vi "CreatePDF XYGraph.vi"(0 "RedPressure":dbl, 1 "BluePressure":dbl, 2 "Print":bool=TRUE, 3 "Blue Graph Refnum":refnum<vi>, 4 "Red Graph Refnum":refnum<vi>) -> ()   [LabVIEW 2013, in "main.lvlib"]
uses:
  main.lvlib
  <userlib>/Exaprom PDF/Controls/Page setup.ctl
  <userlib>/Exaprom PDF/Controls/Page size.ctl
  <userlib>/Exaprom PDF/Controls/Page Orientation.ctl
  <userlib>/Exaprom PDF/Controls/Page Layout Custom.ctl
  <userlib>/Exaprom PDF/Controls/Page margins.ctl
  <userlib>/Exaprom PDF/Controls/PDF Details.ctl
  <userlib>/Exaprom PDF/Controls/Unit.ctl
  <userlib>/Exaprom PDF/Controls/Font cluster.ctl
  <userlib>/Exaprom PDF/Controls/Font size.ctl
  <userlib>/Exaprom PDF/Controls/Font color.ctl
  <userlib>/Exaprom PDF/Controls/Paragraphe cluster.ctl
  <userlib>/Exaprom PDF/Controls/Texte alignement.ctl
  <userlib>/Exaprom PDF/Controls/Line spacing.ctl
  <userlib>/Exaprom PDF/Controls/Image alignment and position.ctl
  <userlib>/Exaprom PDF/Controls/Image aligment.ctl
panel:
  out "error out":errorcluster
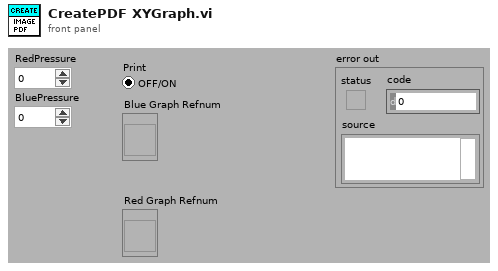
[diagram p1: front panel]
types:
  T1 = typedef "Paragraphe cluster.ctl" = cluster{" Aligment":T2, "Line spacing":T3}
  T2 = typedef "Texte alignement.ctl" = enum16{"Select", "CENTER", "JUSTIFY", "LEFT", "RIGHT"}
  T3 = typedef "Line spacing.ctl" = enum16{"Select", "1.0", "1.5", "2.0"}
  T4 = typedef "Image alignment and position.ctl" = cluster{"Alignment":T5, "X ":sgl, "Y":sgl, "Indentation":sgl}
  T5 = typedef "Image aligment.ctl" = enum16{"Absolute (X,Y) in mm", "Left", "Center", "Right", "Left (textwrap)", "Right (textwrap)"}
  T6 = typedef "Font cluster.ctl" = cluster{"Name":string, "Size":T7, "Color":T8, "Style":cluster{"Bold":bool, "Italic":bool, "Underline":bool, "Strikeout":bool}}
  T7 = typedef "Font size.ctl" = sgl
  T8 = typedef "Font color.ctl" = u32
  T9 = typedef "Unit.ctl" = enum16{"inch", "mm"}
  T10 = typedef "PDF Details.ctl" = cluster{"Title":string, "Subject":string, "Keywords":string, "Author":string, "Creator":string}
  T11 = typedef "Page setup.ctl" = cluster{"Page Size":T12, "Orientation":T13, "Custom Layout":T14, "Margins":T15}
  T12 = typedef "Page size.ctl" = i32
  T13 = typedef "Page Orientation.ctl" = enum16{"Portrait", "Landscape"}
  T14 = typedef "Page Layout Custom.ctl" = cluster{"Width":sgl, "Height":sgl}
  T15 = typedef "Page margins.ctl" = cluster{"Left":sgl, "Right":sgl, "Top":sgl, "Bottom":sgl}
  T16 = typedef "Page dimensions.ctl" = cluster{"Start at page":i32, "Orientation":T13, "widht":sgl, "height":sgl, "Margin left":sgl, "Margin right":sgl, "Margin top":sgl, "Margin bottom":sgl}
  T17 = typedef "Image or Table Caption.ctl" = cluster{"Caption":string, "Separator":string, "Position":enum16{"Above", "Below"}}
  T18 = typedef "Header Footer [ ].ctl" = T19[]
  T19 = typedef "Header Footer cluster.ctl" = cluster{"Start page":i32, "Type":T20, "Alignment":T21, "Vertical Alignement":T22, "Image (%)":sgl, "Page #":T23, "Text":string, "Path":string, "Font":T6, "Font refnum":refnum<k24>, "Line":cluster{"Line":T24, "Thickness (points)":sgl, "Colour":T8}}
  T20 = typedef "Header Footer Type.ctl" = enum16{"Select", "Text", "Text + hyperlink", "Page number", "Image", "Image + hyperlink"}
  T21 = typedef "Header footer horiz alignment.ctl" = enum16{"Left", "Center", "Right"}
  T22 = typedef "Cell Vertical alignment.ctl" = enum16{"TOP", "MIDDLE", "BOTTOM"}
  T23 = typedef "Page number.ctl" = cluster{"Text 1":string, "Text 2":string, "Text 3":string}
  T24 = typedef "Header Footer Line.ctl" = enum16{"No line", "Horizontal line"}
  T25 = typedef "Watermark cluster2.ctl" = cluster{"Show? (F)":bool, "Type":enum16{"Image", "Text"}, "Opacity (%)":sgl, "Rotate(°)":sgl, "Position":cluster{"Position":T26, "X":sgl, "Y":sgl}, "Image path":path, "Scaled(%)":sgl, "Image refnum":refnum<k24>, "Text":string, "Font":cluster{"Name":string, "Size":T7, "Color":T8}, "Font refnum":refnum<k24>, "Alignment":T21, "Automatic":bool}
  T26 = typedef "Watermark Position.ctl" = enum16{"Absolute", "Center (page)", "Center (text section)"}
  T27 = typedef "System Fonts.ctl" = cluster{"Font name [ ]":string[], "Font and file names [ ]":cluster{"Font name":string, "File name":string}[]}
  T28 = cluster{"Document":refnum<k24>, "Writer":refnum<k24>, "Default Font":refnum<k24>, "Default Font cluster":T6, "Path":path, "Unit (default = mm)":T9, "Paragraphe cluster":T1, "Pages dimensions [ ]":T16[], "Captions":cluster{"Image":T17, "Image counter":u16, "Table":T17, "Table counter":u16, "Font":T6}, "Header":T18, "Footer":T18, "Watermark ":T25, "Actual VI name":string, "System Fonts":T27}
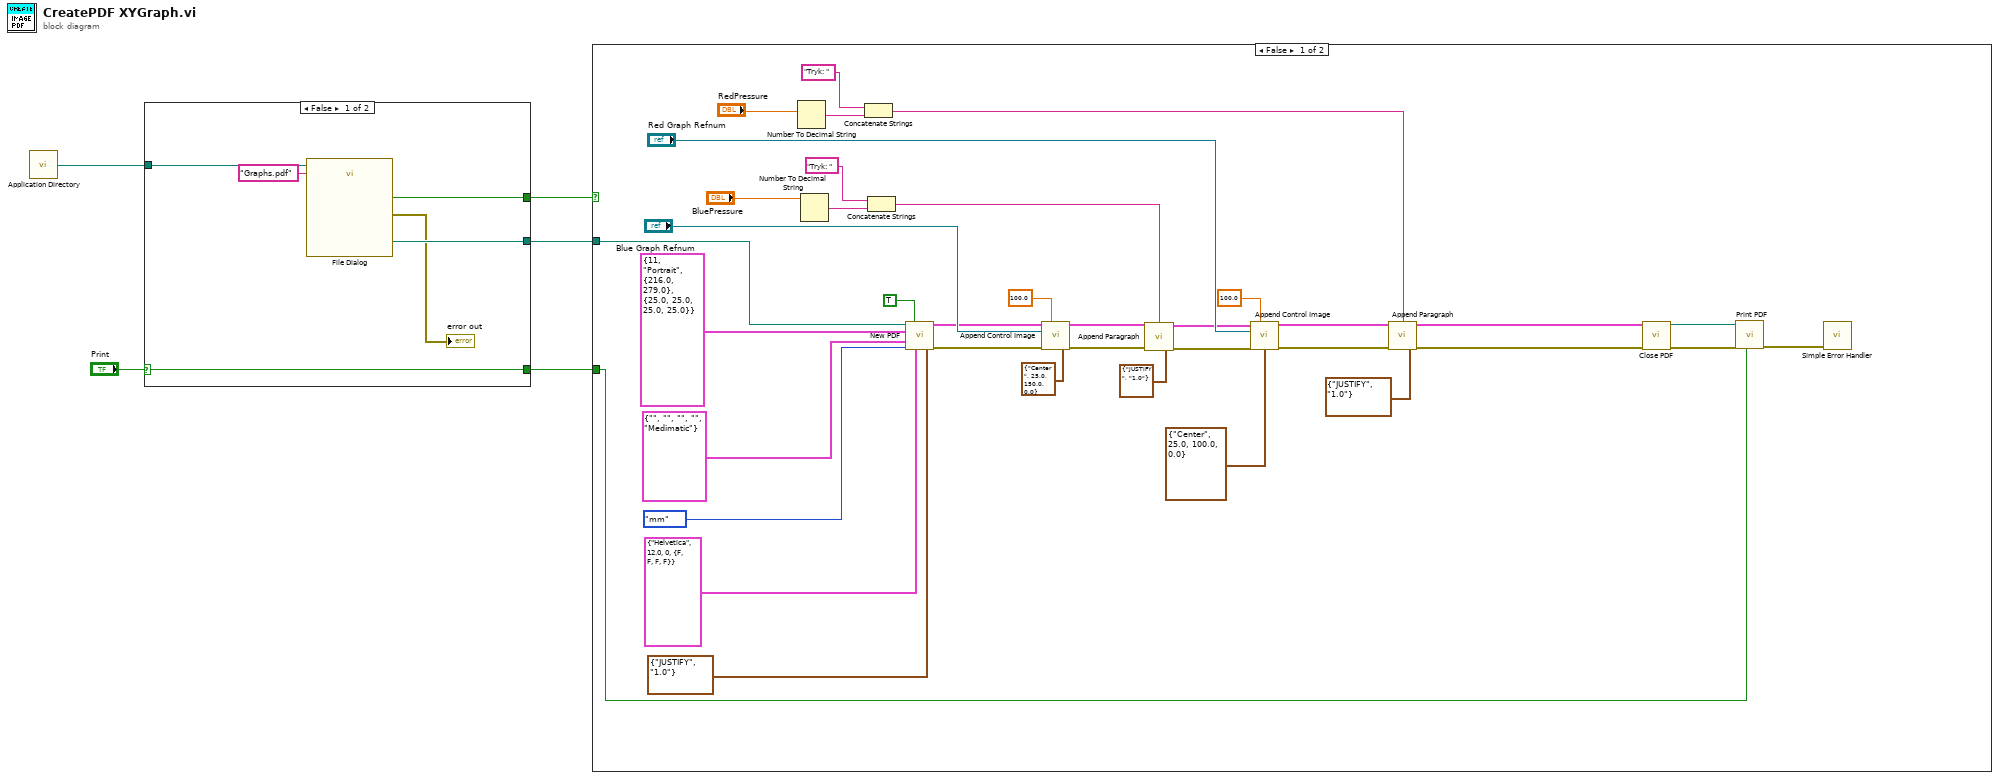
[diagram p0: block diagram]
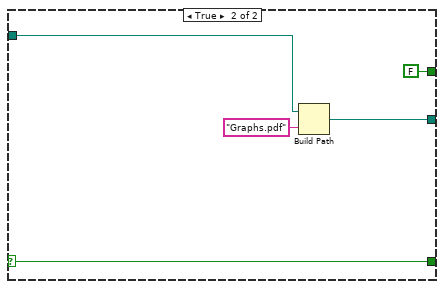
[diagram p2: hidden frame]
diagram:
  n1 = call <vilib>:"Application Directory.vi"() -> ("Application Directory"=w4:path)
  n2 = case shown="False" "Print" {
    selector: "Print" -> [w6 w16]
    tunnel: [w11 w14] -> w5
    tunnel: w4 -> [w10 w13]
    tunnel: [w8 FALSE ("cancelled")] -> w3
    tunnel: [w6 w16] -> w1
    frame False {
      n3 = call "File Dialog"("start path"=w10, "default name"="Graphs.pdf") -> ("selected path"=w11:path, "cancelled"=w8:bool, "error out"=→"error out":errorcluster)  [unwired: 10 in, 1 out]
    }
    frame True {
      n4 = Build Path(base path=w13, name or relative path="Graphs.pdf") -> (appended path=w14:path)
    }
  }
  n5 = case shown="False" w3 {
    tunnel: w5 -> [w21 _]
    tunnel: w1 -> [w19 _]
    frame False {
      n6 = Number To Decimal String(number="RedPressure") -> (decimal integer string=w30:string)  [unwired: 1 in]
      n7 = Number To Decimal String(number="BluePressure") -> (decimal integer string=w34:string)  [unwired: 1 in]
      n8 = Concatenate Strings("Tryk: ", w30) -> (w29:string)
      n9 = Concatenate Strings("Tryk: ", w34) -> (w33:string)
      n10 = call <userlib>:"New PDF.vi"("PDF Path"=w21, "Overwrite?"=TRUE, "Page Setup"=T11 {"Page Size"=11, "Orientation"=enum."Portrait", "Custom Layout"={"Width"=216.0, "Height"=279.0}, "Margins"={"Left"=25.0, "Right"=25.0, "Top"=25.0, "Bottom"=25.0}}, "PDF Details"=T10 {"Title"="", "Subject"="", "Keywords"="", "Author"="", "Creator"="Medimatic"}, "Unit (default = mm)"=Unit."mm", "Default Font"=T6 {"Name"="Helvetica", "Size"=12.0, "Color"=0, "Style"={"Bold"=FALSE, "Italic"=FALSE, "Underline"=FALSE, "Strikeout"=FALSE}}, "Default Paragraph"=T1 {" Aligment"=enum."JUSTIFY", "Line spacing"=enum."1.0"}) -> ("PDF Report"=w49:T28, "error out"=w50:errorcluster)  [unwired: 7 in]
      n11 = call <userlib>:"Append Control Image.vi"("PDF Report IN"=w49, "Scale (%)"=sgl 100.0, "Ctrl reference"="Blue Graph Refnum", "error in (no error)"=w50, "Position and indentation"=T4 {"Alignment"=enum."Center", "X "=25.0, "Y"=150.0, "Indentation"=0.0}) -> ("PDF Report OUT"=w40:T28, "error out"=w39:errorcluster)  [unwired: 9 in]
      n12 = call <userlib>:"Append Paragraph.vi"("PDF Report"=w40, "Text"=w33, "error in (no error)"=w39, "Paragraph properties"=T1 {" Aligment"=enum."JUSTIFY", "Line spacing"=enum."1.0"}) -> ("PDF Report duplicate"=w38:T28, "error out"=w37:errorcluster)  [unwired: 10 in]
      n13 = call <userlib>:"Append Control Image.vi"("PDF Report IN"=w38, "Scale (%)"=sgl 100.0, "Ctrl reference"="Red Graph Refnum", "error in (no error)"=w37, "Position and indentation"=T4 {"Alignment"=enum."Center", "X "=25.0, "Y"=100.0, "Indentation"=0.0}) -> ("PDF Report OUT"=w28:T28, "error out"=w27:errorcluster)  [unwired: 9 in]
      n14 = call <userlib>:"Append Paragraph.vi"("PDF Report"=w28, "Text"=w29, "error in (no error)"=w27, "Paragraph properties"=T1 {" Aligment"=enum."JUSTIFY", "Line spacing"=enum."1.0"}) -> ("PDF Report duplicate"=w25:T28, "error out"=w26:errorcluster)  [unwired: 10 in]
      n15 = call <userlib>:"Close PDF.vi"("PDF Report"=w25, "error in (no error)"=w26) -> ("Path"=w24:path, "error out"=w23:errorcluster)  [unwired: 12 in]
      n16 = call <userlib>:"Print PDF.vi"("Print (T)"=w19, "error in (no error)"=w23, "path"=w24) -> ("error out"=w22:errorcluster)  [unwired: 6 in]
      n17 = call <vilib>:"Simple Error Handler.vi"("error in (no error)"=w22) -> ()  [unwired: 4 in, 5 out]
    }
    frame True {
    }
  }
